vi "Fake Recreate Client.vi"(8 "error in":errorcluster, 11 "grpc client id in":T1) -> (0 "error out":errorcluster, 3 "grpc client id out":T1)   [LabVIEW 2020, in "MeasurementServerTests.lvlib" / "gRPC Utilities Tests.lvlib"]
uses:
  gRPC Utilities Tests.lvlib
  <vilib>/gRPC/LabVIEW gRPC Library/Shared/grpcId.ctl
  <vilib>/gRPC/LabVIEW gRPC Library/grpc-lvsupport-release.lvlib
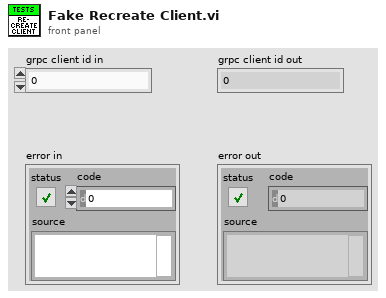
[diagram p1: front panel]
types:
  T1 = typedef "grpc-lvsupport-release.lvlib/grpcId.ctl" = u64
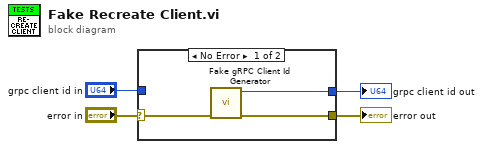
[diagram p0: block diagram]
diagram:
  n1 = case shown="No Error" "error in" {
    selector: "error in" -> [w7 w8]
    tunnel: [w6 w8] -> w3
    tunnel: [w5 _] -> w2
    tunnel: "grpc client id in" -> [_ _]
    frame No Error {
      n2 = call "Fake gRPC Client Id Generator.vi"("error in"=w7) -> ("error out"=w6:errorcluster, "client id"=w5:u64)  [unwired: 9 in]
    }
    frame Error {
    }
  }
  "error out" <- w3
  "grpc client id out" <- w2
